vi "PSUTI_Toolbar Buttons.vi"() -> ()   [LabVIEW 2016]
panel:
  in  "Delete 4":bool
  in  "Add 3":bool
  in  "Paste":bool
  in  "Copy":bool
  in  "LogIn 2":bool
  in  "Quit":bool
  in  "Hide Navigator":bool
  in  "Exp Main":bool
  in  "Person Main":bool
  in  "LogIn":bool
  in  "OpenFile":bool
  in  "Check Data":bool
  in  "Config Plan":bool
  in  "Pack":bool
  in  "Print":bool
  in  "SetTime 2":bool
  in  "SetTime":bool
  in  "History":bool
  in  "Delete 3":bool
  in  "Add 2":bool
  in  "Delete 2":bool
  in  "Draw Process":bool
  in  "Search":bool
  in  "布尔":bool
  in  "Device Oper 2":cluster{"Export":bool, "Import":bool}
  in  "Stop Test":bool
  in  "?":bool
  in  "Start Test":bool
  in  "Commit":bool
  in  "More Log":bool
  in  "Export Word":bool
  in  "Export Excel":bool
  in  "Device Oper":cluster{"Export":bool, "Import":bool}
  in  "Left":bool
  in  "Right":bool
  in  "Cancel":bool
  in  "Ok":bool
  in  "Personal Choose":bool
  in  "Device Choose":bool
  in  "Export Report":bool
  in  "Open":bool
  in  "Shift Out Function":bool
  in  "Add Function":bool
  in  "Complete Tag":bool
  in  "Confirm":bool
  in  "Generation":bool
  in  "Revert":bool
  in  "Ignore":bool
  in  "Shift Out":bool
  in  "Shift In":bool
  in  "Export":bool
  in  "Import":bool
  in  "Add":bool
  in  "Save":bool
  in  "Delete":bool
  in  "Assess":bool
  in  "Inter":bool
  in  "Download":bool
  in  "Upload":bool
  in  "Edit":bool
  in  "Import Picture":bool
  in  "New":bool
  in  "Update":bool
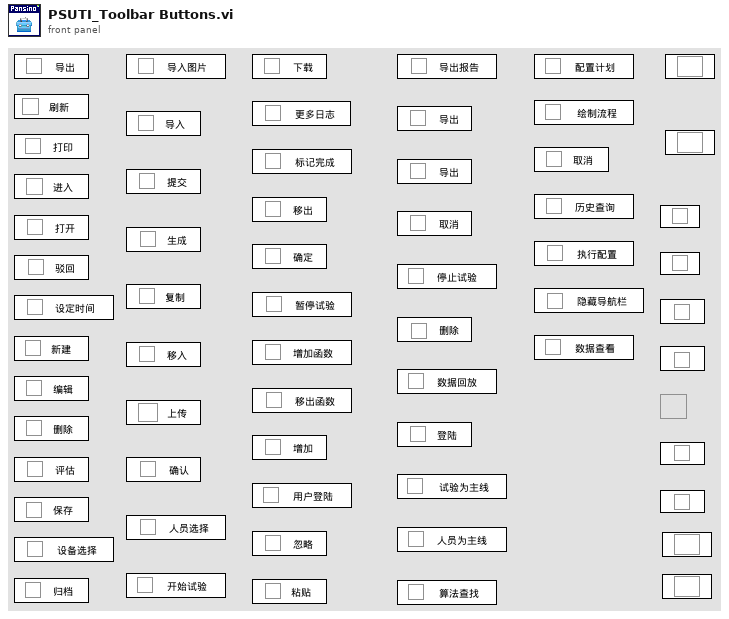
[diagram p1: front panel]
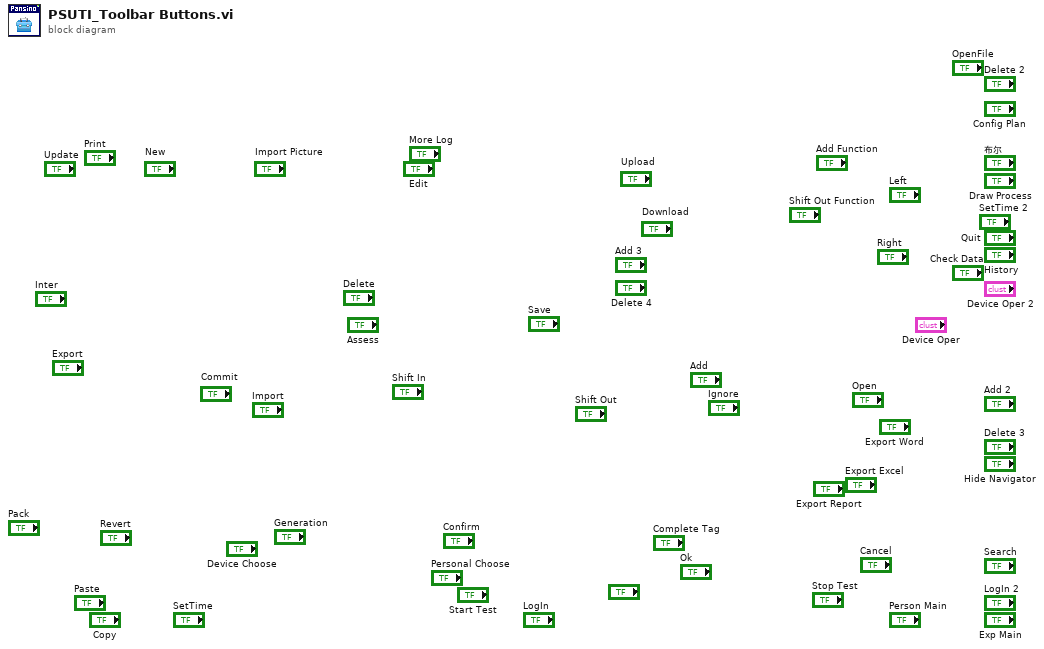
[diagram p0: block diagram]
diagram:
